vi "Main_02a.vi"() -> ()   [LabVIEW 2023]
uses:
  ENUM Color.ctl
  <vilib>/Utility/miscctls.llb/LVMapReplaceAction.ctl
  <vilib>/Utility/error.llb/Trim Whitespace One-Sided.vi
panel:
  out "Map":map{T1, i32}(c390)
  out "Answer":i32
  in  "Puzzle":string="Game 1: 1 green, 1 blue, 1 red; 3 green, 1 blue, 1 red; 4 green, 3 blue, 1 red; 4 green, 2 blue, 1 red; 3 blue, 3 green\nGame 2: 9 blue, 7 red; 5 blue, 6 green, 1 red; 2 blue, 10 red, 9 green; 3 green, 14 red, 5 blue; 8 red, 3 blue, 4 green; 8 green, 14 blue, 10 red\nGame 3: 11 green, 8 blue, 7 red; 3 green, 4 red, 9 blue; 3 red, 4 green, 8 blue; 11 green, 1 red, 16 blue\nGame 4: 3 blue, 20 green, 2 red; 1 green, 3 red, 3 blue; 1 blue, 9 green; 4 red, 17 green; 12 green, 3 red\nGame 5: 2 red, 1 blue, 4 green; 6 blue, 2 green; 2 red, 5 green\nGame 6: 1 green, 7 red; 1 blue, 3 green, 1 red; 1 blue, 2 red, 2 green; 1 blue, 1 green, 2 red; 3 red; 8 red, 1 green, 1 blue\nGame 7: 13 green, 5 blue, 1 red; 9 green, 6 blue; 11 green, 2 blue, 2 red\nGame 8: 2 red, 11 green, 6 blue; 5 green, 3 blue; 3 blue, 3 green, 5 red; 5 blue, 9 green, 1 red\nGame 9: 3 blue, 5 green, 8 red; 4 green, 19 blue, 4 red; 4 red, 17 blue\nGame 10: 2 green, 8 red, 4 blue; 1 green, 5 red, 9 blue; 3 green, 2 red, 4 blue; 2 green, 5 red, 2 blue; 6 green, 4 blue; 10 blue, 8 green, 8 red\nGame 11: 3 green, 1 blue, 9 red; 2 blue, 1 red, 9 green; 1 blue, 9 green, 7 red; 8 red, 6 green\nGame 12: 5 green; 8 green, 7 red, 1 blue; 8 blue, 8 green, 14 red; 6 red, 14 green; 14 green, 3 red, 8 blue\nGame 13: 7 red, 2 green, 4 blue; 5 red, 3 blue, 8 green; 10 green, 1 red, 4 blue; 7 green, 1 red, 13 blue; 11 green, 12 blue, 2 red\nGame 14: 9 green, 4 red; 7 green, 4 blue, 5 red; 2 red, 2 green; 3 green, 2 red, 8 blue; 7 green, 6 red, 8 blue\nGame 15: 19 blue, 1 green; 1 red, 5 blue; 3 green, 8 blue; 1 red, 13 blue, 3 green\nGame 16: 8 red, 11 blue, 3 green; 14 green, 1 red, 12 blue; 6 green, 1 red, 6 blue; 1 red, 6 blue, 17 green; 2 green, 8 blue, 3 red\nGame 17: 3 red, 1 blue; 1 blue, 2 red, 1 green; 1 red; 3 red, 2 green\nGame 18: 8 green, 2 red; 1 blue, 6 red; 8 green, 7 red, 2 blue; 1 red; 6 green, 1 blue, 3 red\nGame 19: 4 blue, 2 green; 4 green, 18 blue, 2 red; 14 green, 4 blue; 1 red, 3 blue, 18 green; 11 blue, 3 red; 14 green, 4 red, 6 blue\nGame 20: 7 blue; 1 blue, 6 green, 1 red; 1 red, 3 blue, 10 green; 7 green, 4 blue, 1 red; 6 green, 6 blue, 1 red; 1 red, 5 blue, 17 green\nGame 21: 11 blue, 9 red; 8 red, 2 blue; 2 red, 11 blue, 2 green\nGame 22: 4 green, 9 blue, 2 red; 2 blue, 8 green; 2 green, 2 red, 6 blue\nGame 23: 7 green, 7 blue; 6 blue, 11 green; 1 red, 14 green; 15 green, 4 blue, 1 red; 1 red, 5 blue, 3 green; 1 red, 1 blue, 13 green\nGame 24: 5 green, 2 red, 2 blue; 1 blue, 3 green, 2 red; 2 blue, 7 green, 3 red\nGame 25: 16 red, 8 green; 2 red, 3 blue; 10 green, 5 red, 4 blue; 9 red, 7 green; 7 red, 6 blue\nGame 26: 3 red, 1 green; 5 red, 1 blue, 10 green; 8 red, 5 green\nGame 27: 3 red, 2 blue; 6 red, 8 green; 5 green, 13 red, 2 blue; 4 red, 1 blue, 8 green; 14 red, 1 blue, 3 green; 2 red, 1 green, 2 blue\nGame 28: 9 red, 10 blue; 9 red, 9 blue; 1 green, 6 red, 4 blue; 12 blue, 3 green, 2 red; 2 green, 12 red, 8 blue\nGame 29: 4 red, 15 blue; 5 blue, 3 green, 6 red; 1 green, 9 blue, 1 red; 5 green, 8 red, 1 blue\nGame 30: 4 green, 2 blue, 10 red; 1 red, 5 green, 6 blue; 15 red, 2 blue; 5 green, 10 red, 8 blue\nGame 31: 6 green, 2 blue, 2 red; 5 green, 6 red, 6 blue; 3 blue, 5 red, 1 green; 4 green, 6 red, 9 blue; 4 red; 3 green, 1 red, 3 blue\nGame 32: 8 green, 17 red, 17 blue; 11 red, 6 green, 13 blue; 14 red, 1 green, 1 blue; 1 green, 17 red, 4 blue; 5 green, 14 red, 15 blue; 15 blue, 8 green\nGame 33: 2 red, 14 blue; 3 blue, 17 red, 4 green; 9 blue, 8 red; 5 red, 2 blue; 4 green, 16 red, 5 blue; 15 blue, 6 green, 17 red\nGame 34: 12 green, 2 red, 1 blue; 3 blue, 9 red, 13 green; 2 blue, 17 green, 6 red; 6 green, 4 red, 3 blue; 2 red, 1 blue; 7 green, 3 blue, 7 red\nGame 35: 4 blue, 5 red, 5 green; 6 green, 12 red, 6 blue; 3 green, 18 red, 2 blue; 13 red, 6 green, 9 blue; 3 green, 10 blue, 17 red; 1 green, 3 blue, 16 red\nGame 36: 4 green, 3 blue, 1 red; 3 green, 3 red, 10 blue; 1 red, 8 green, 8 blue; 3 blue, 1 red; 2 red, 2 blue, 14 green\nGame 37: 16 blue, 1 green; 9 blue; 7 red, 13 blue\nGame 38: 6 green, 8 red, 3 blue; 5 blue, 4 green, 6 red; 5 blue, 4 green; 5 red, 3 green, 1 blue; 6 green, 4 blue, 15 red\nGame 39: 10 blue, 4 green; 1 blue, 7 green, 5 red; 8 red, 2 blue\nGame 40: 2 blue, 2 green, 6 red; 8 green, 4 red, 2 blue; 4 blue, 12 green, 6 red\nGame 41: 4 green, 2 blue, 11 red; 6 red, 11 green; 4 blue, 2 red, 19 green; 3 green, 2 blue, 1 red\nGame 42: 2 blue, 2 green, 4 red; 1 red, 4 blue, 8 green; 5 red, 2 blue, 15 green; 10 green, 5 red, 1 blue; 10 green, 1 blue; 2 blue\nGame 43: 10 red, 19 green, 11 blue; 11 green, 1 red, 2 blue; 13 red, 6 blue, 3 green; 12 red, 10 green; 5 red, 19 green, 8 blue; 2 red, 10 green, 3 blue\nGame 44: 7 blue, 8 red; 1 green, 12 red; 19 red, 3 green, 5 blue\nGame 45: 12 red; 2 green, 5 red, 3 blue; 10 green, 2 blue, 4 red; 10 green, 7 red\nGame 46: 4 blue, 4 red, 2 green; 7 green, 6 blue; 6 blue, 1 red, 4 green\nGame 47: 4 green, 8 red, 1 blue; 4 green, 1 blue, 11 red; 14 red, 3 blue, 10 green; 15 green, 2 blue, 7 red\nGame 48: 6 blue, 3 green, 1 red; 15 blue, 11 red, 3 green; 17 blue, 14 red; 2 green, 13 red; 5 red, 2 green, 4 blue\nGame 49: 7 blue, 1 green; 8 red, 2 blue, 1 green; 1 red, 1 green, 2 blue; 3 red, 2 blue, 1 green\nGame 50: 13 red, 2 green, 2 blue; 13 red, 6 green, 1 blue; 12 red, 8 green; 1 red, 3 green; 13 red; 2 blue, 11 red, 2 green\nGame 51: 7 green, 4 blue, 2 red; 3 red, 7 green, 5 blue; 10 green, 2 blue; 14 green, 3 red, 4 blue; 2 blue, 2 red, 10 green\nGame 52: 7 blue, 10 red; 7 red, 4 blue, 8 green; 12 red, 4 blue, 7 green; 7 green, 7 red; 17 green, 11 blue, 6 red; 8 green, 8 red, 18 blue\nGame 53: 6 green, 2 red; 10 red, 13 green; 2 blue, 3 green, 5 red; 4 red, 4 green; 8 green, 1 red; 13 green, 2 blue, 10 red\nGame 54: 5 red, 9 green, 5 blue; 6 red, 15 green, 10 blue; 8 blue, 3 green, 1 red; 12 blue, 3 red, 13 green\nGame 55: 10 green, 4 red, 2 blue; 2 green, 1 red, 2 blue; 2 blue, 4 red, 8 green; 5 blue, 3 green\nGame 56: 7 green, 9 red, 2 blue; 4 red, 1 blue, 3 green; 3 red, 4 blue, 6 green; 7 green, 2 red; 5 blue, 2 red, 3 green; 7 green, 7 red, 5 blue\nGame 57: 11 blue, 5 green, 6 red; 18 red, 15 green, 10 blue; 5 green, 14 red, 6 blue; 1 green, 11 red, 7 blue; 11 blue, 7 red, 12 green\nGame 58: 9 red, 6 blue, 6 green; 6 blue, 12 red, 3 green; 8 red, 1 blue, 20 green; 3 green, 3 red, 15 blue; 4 blue, 15 green, 3 red\nGame 59: 18 red, 4 blue, 7 green; 11 blue, 19 red, 7 green; 10 red, 9 blue, 1 green; 8 red, 12 green, 4 blue; 6 green, 5 blue, 12 red; 2 blue, 14 green, 2 red\nGame 60: 1 blue, 9 green, 6 red; 1 red, 1 blue, 13 green; 15 green, 4 red; 1 blue, 2 red, 15 green\nGame 61: 9 green, 3 red, 2 blue; 1 green, 5 blue, 10 red; 17 red, 9 green, 5 blue; 10 red, 5 green, 5 blue\nGame 62: 4 red, 2 green; 2 red; 5 red, 2 green, 2 blue; 3 green, 1 blue; 2 blue, 3 red, 3 green\nGame 63: 4 red, 6 blue, 2 green; 3 green, 1 red, 5 blue; 7 blue, 5 green\nGame 64: 8 blue, 12 red; 1 green, 6 red, 14 blue; 12 red, 13 blue\nGame 65: 2 red, 8 green; 1 blue, 2 red, 5 green; 2 blue, 3 green; 1 green, 1 red\nGame 66: 6 red, 8 blue, 2 green; 6 blue, 7 green; 7 green, 11 blue; 5 green, 4 red, 10 blue; 5 blue, 4 green; 6 blue, 6 green, 5 red\nGame 67: 12 green, 4 red; 2 blue, 11 green, 6 red; 9 red, 2 green, 6 blue; 2 red, 8 blue, 18 green; 17 green, 7 blue, 6 red; 12 blue, 9 green\nGame 68: 3 red, 9 blue, 1 green; 3 green, 11 blue; 12 blue, 9 red; 6 red, 13 green, 8 blue\nGame 69: 3 red, 8 green, 3 blue; 6 green, 3 red; 11 green, 3 blue; 4 red, 3 green; 7 green, 4 blue, 6 red; 1 red, 2 blue\nGame 70: 6 green, 4 blue; 7 red, 9 green, 14 blue; 12 red; 9 green, 10 red; 6 green, 16 blue, 8 red\nGame 71: 4 blue, 6 red, 9 green; 6 green, 2 red; 8 green, 4 blue, 2 red; 1 red, 3 blue, 8 green; 9 green, 3 red, 3 blue; 4 red, 6 green\nGame 72: 3 red, 3 green, 3 blue; 4 red, 1 green, 3 blue; 2 red, 2 green, 1 blue\nGame 73: 7 green, 6 red, 7 blue; 2 green, 4 blue; 2 blue, 15 green, 4 red; 1 blue, 4 green, 2 red; 7 blue, 14 green\nGame 74: 4 green, 2 red, 2 blue; 9 blue, 13 green, 4 red; 10 green, 12 blue, 7 red; 4 blue, 8 green, 7 red\nGame 75: 3 red, 3 green; 3 green, 12 red; 18 red, 2 blue; 3 green, 9 red, 1 blue; 14 red, 1 green; 15 red\nGame 76: 1 blue, 7 red, 8 green; 3 blue, 4 red, 1 green; 6 green, 6 red\nGame 77: 2 green, 8 red; 5 green, 11 red, 1 blue; 5 red, 2 blue, 2 green; 6 red, 5 green, 2 blue; 11 red, 2 green, 1 blue; 2 red, 8 green, 2 blue\nGame 78: 1 blue, 4 red, 10 green; 13 green, 4 red, 9 blue; 12 green, 6 blue, 3 red; 5 blue, 8 green, 6 red\nGame 79: 9 red, 1 blue, 17 green; 9 green, 6 red; 15 green, 1 blue, 9 red; 1 blue, 8 red, 12 green; 11 green, 1 blue, 1 red\nGame 80: 3 red, 3 blue, 1 green; 1 blue, 8 green; 10 green, 16 blue\nGame 81: 15 blue, 2 red; 1 red, 8 blue; 2 green, 7 red, 11 blue; 19 blue, 8 red, 2 green; 20 red, 19 blue\nGame 82: 3 red, 17 blue, 9 green; 10 red, 2 green, 17 blue; 13 red, 3 blue, 10 green; 11 red, 10 green, 18 blue; 1 green, 12 blue, 9 red; 3 red, 10 blue, 8 green\nGame 83: 4 green, 2 blue, 14 red; 7 red, 2 blue, 7 green; 16 red, 7 green; 16 red, 2 green; 3 blue, 4 green, 15 red; 6 red, 1 blue, 4 green\nGame 84: 4 blue, 1 green, 2 red; 7 blue, 6 red; 1 blue, 4 red, 3 green\nGame 85: 5 blue, 1 red, 4 green; 14 blue, 7 green; 9 blue, 1 red, 7 green; 15 blue, 9 green; 8 blue, 6 green, 1 red\nGame 86: 12 red, 12 blue, 7 green; 16 red, 11 green, 4 blue; 14 blue, 8 green, 8 red; 2 blue, 15 red, 6 green; 1 green, 6 red, 5 blue; 11 blue, 9 green\nGame 87: 4 blue, 2 green, 6 red; 8 red, 3 green, 5 blue; 10 red, 1 green; 1 green, 3 blue, 1 red\nGame 88: 2 green, 2 red, 4 blue; 4 blue, 4 green, 12 red; 2 green, 3 blue, 4 red; 2 green, 2 blue, 12 red; 4 blue, 8 red, 2 green\nGame 89: 13 blue, 1 red, 5 green; 8 green, 16 blue, 5 red; 12 green, 2 red, 18 blue\nGame 90: 7 red, 11 blue, 1 green; 8 green, 13 blue; 7 green, 16 blue; 5 green, 13 red, 11 blue; 5 blue, 10 green, 3 red\nGame 91: 1 blue; 1 blue, 3 green; 1 green, 2 red\nGame 92: 16 red, 4 blue, 14 green; 15 red, 7 blue, 13 green; 7 green, 13 red, 8 blue; 4 blue, 9 red, 5 green; 6 red, 7 blue, 8 green; 14 green, 7 red, 10 blue\nGame 93: 2 red, 6 blue, 7 green; 8 green, 3 red, 10 blue; 1 green, 4 red; 2 red, 2 green; 8 blue, 7 green\nGame 94: 2 green, 3 blue, 5 red; 10 blue; 1 green, 7 red; 3 blue, 1 green, 12 red\nGame 95: 13 blue, 5 red; 9 blue, 3 red, 7 green; 10 green, 4 red, 12 blue; 14 blue; 7 green, 2 blue, 1 red\nGame 96: 5 red, 2 blue; 4 red; 1 green, 2 blue\nGame 97: 9 red, 10 green, 3 blue; 2 green, 15 red, 1 blue; 2 blue, 16 green, 16 red; 8 green, 14 red; 16 red\nGame 98: 18 green, 16 red, 1 blue; 3 red, 2 blue, 20 green; 1 blue, 20 green, 14 red; 14 red, 2 green\nGame 99: 7 red, 9 green, 5 blue; 6 blue, 1 green; 4 green, 5 blue, 1 red; 8 green, 6 red, 7 blue; 1 blue, 2 red, 9 green\nGame 100: 10 blue, 2 red; 7 green, 20 blue, 9 red; 8 red, 6 green, 2 blue"
  in  "Example":string="Game 1: 3 blue, 4 red; 1 red, 2 green, 6 blue; 2 green\nGame 2: 1 blue, 2 green; 3 green, 4 blue, 1 red; 1 green, 1 blue\nGame 3: 8 green, 6 blue, 20 red; 5 blue, 4 red, 13 green; 5 green, 1 red\nGame 4: 1 green, 3 red, 6 blue; 3 green, 6 red; 3 green, 15 blue, 14 red\nGame 5: 6 red, 1 blue, 3 green; 2 blue, 1 red, 2 green"
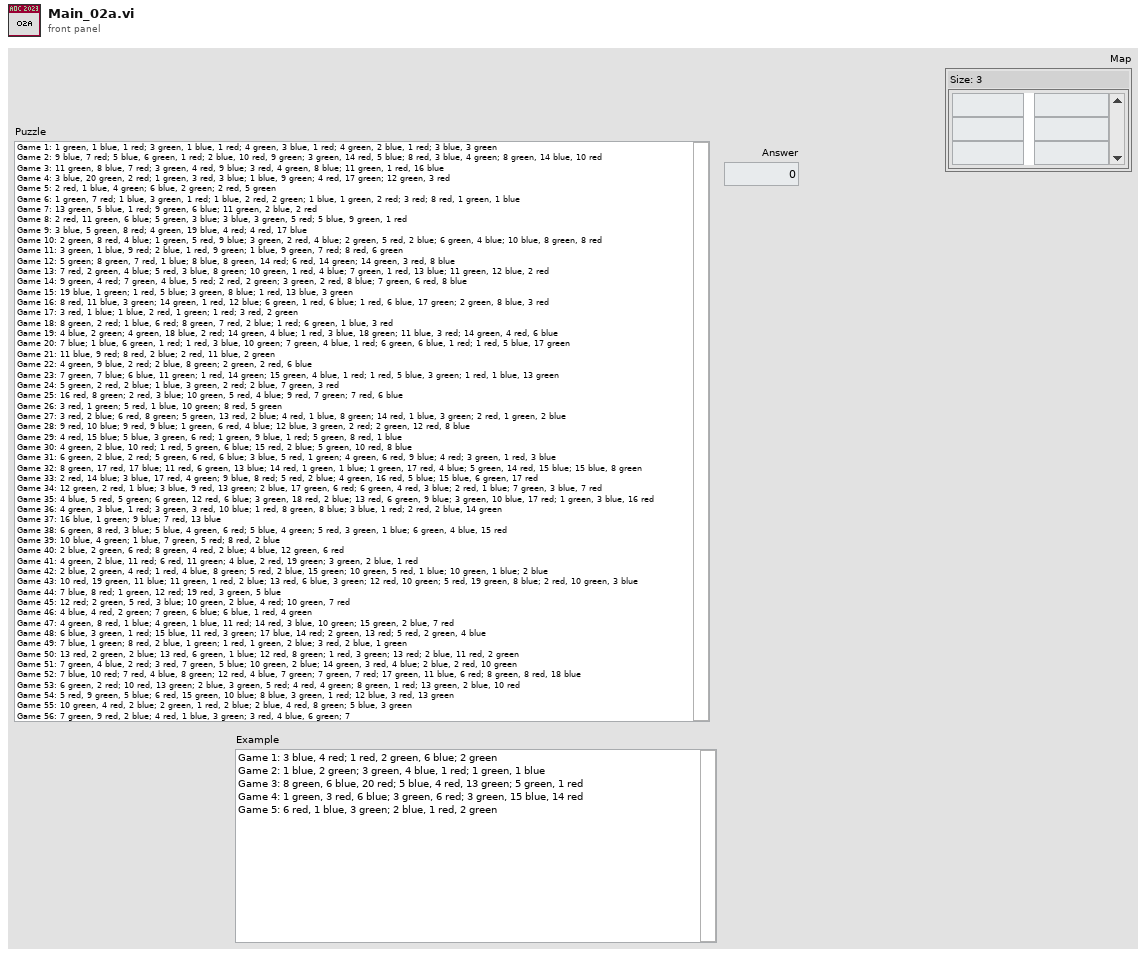
[diagram p1: front panel]
types:
  T1 = typedef "ENUM Color.ctl" = enum16{"red", "green", "blue"}
  T2 = typedef "LVMapReplaceAction.ctl" = enum32{"Modify Entry only if found", "Add or Modify Entry", "Delete Entry"}
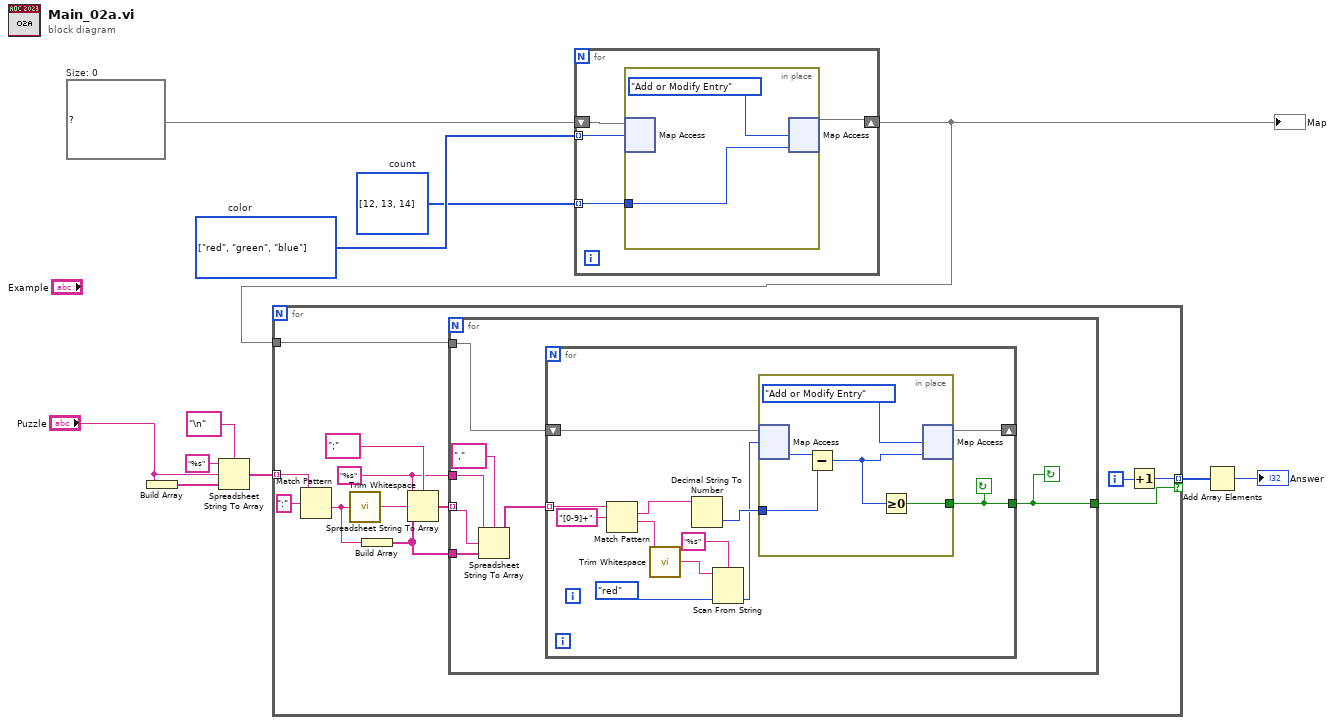
[diagram p0: block diagram]
diagram:
  w7 = i32[] [12, 13, 14]  # count
  w8 = T1[] [enum."red", enum."green", enum."blue"] items=["red", "green", "blue"]  # color
  w5 = map{T1, i32} {}  # Size: 0
  n1 = Build Array("Puzzle") -> (w11:string[])
  n2 = Spreadsheet String To Array(delimiter (Tab)="\n", format string="%s", spreadsheet string="Puzzle", array type (2D Dbl)=w11) -> (array=w6:string[])
  n3 = for {
    shift-right: [w14] -> w4
    shift-left: w5 -> [w15]
    tunnel: w8 -> [w13] mode=indexing
    tunnel: w7 -> [w12] mode=indexing
    n4 = in-place {
      in-place-border: w12 -> [w16]
      n5 = in-place-map #1(w15, w13) -> ()  [unwired: 1 in, 2 out]
      n6 = in-place-map #1(w16, LVMapReplaceAction."Add or Modify Entry" ("action")) -> (w14:map{T1, i32})  [unwired: 2 out]
    }
  }
  "Map" <- w4
  n7 = for {
    tunnel: w6 -> [w29] mode=indexing
    tunnel: w4 -> [w23]
    tunnel: [w19] -> w3 mode=indexing if=w18
    i -> [w20]
    w21 = "%s" ("format string")
    n8 = Match Pattern(string=w29, regular expression=":") -> (after substring=w25:string)  [unwired: 1 in, 3 out]
    n9 = call <vilib>:"Trim Whitespace.vi"("string"=w25) -> ("trimmed string"=w27:string)  [unwired: 1 in]
    n10 = Build Array(w25) -> (w22:string[])
    n11 = Spreadsheet String To Array(delimiter (Tab)=";", format string=w21, spreadsheet string=w27, array type (2D Dbl)=w22) -> (array=w24:string[])
    n12 = for {
      tunnel: w24 -> [w32] mode=indexing
      tunnel: [w30] -> w18
      tunnel: w23 -> [w36]
      tunnel: w22 -> [w34]
      tunnel: w21 -> [w31]
      stop <- w30 continue-if-true
      n13 = Spreadsheet String To Array(delimiter (Tab)=",", format string=w31, spreadsheet string=w32, array type (2D Dbl)=w34) -> (array=w33:string[])
      n14 = for {
        tunnel: [w37] -> w30
        tunnel: w33 -> [w38] mode=indexing
        shift-right: [w40] -> _
        shift-left: w36 -> [w41]
        stop <- w37 continue-if-true
        n15 = Match Pattern(string=w38, regular expression="[0-9]+") -> (match substring=w47:string, after substring=w48:string)  [unwired: 1 in, 2 out]
        n16 = call <vilib>:"Trim Whitespace.vi"("string"=w48) -> ("trimmed string"=w45:string)  [unwired: 1 in]
        n17 = Decimal String To Number(string=w47) -> (number=w42:i32)  [unwired: 2 in, 1 out]
        n18 = Scan From String(format string="%s", input string=w45, default 1=ENUM_Color."red" ("Enum")) -> (output 1=w39:T1)  [unwired: 2 in, 3 out]
        n19 = in-place {
          in-place-border: w42 -> [w51]
          in-place-border: [w49] -> w37
          n20 = in-place-map #2(w41, w39) -> (w52:i32)  [unwired: 1 in, 1 out]
          n21 = Subtract(x=w52, y=w51) -> (x-y=w50:i32)
          n22 = Greater Or Equal To 0?(x=w50) -> (x >= 0?=w49:bool)
          n23 = in-place-map #2(w50, LVMapReplaceAction."Add or Modify Entry" ("action")) -> (w40:map{T1, i32})  [unwired: 2 out]
        }
      }
    }
    n24 = Increment(x=w20) -> (x+1=w19:i32)
  }
  n25 = Add Array Elements(numeric array=w3) -> (sum=→"Answer":i32)
